vi "Begin.vi"(8 "error in":errorcluster) -> (0 "error out":errorcluster)   [LabVIEW 2015]
doc: "Called before other user functions, this VI is expected to open initial I/O refnums, load in file data, and do all program initialization. Notice that the <B>error out</B> terminal is simply used for data flow. Wiring it to other structures or subVIs ensures that this VI runs first."
uses:
  <vilib>/Rock Robotics/SystemInterfaces/DIO/FPGA_DIOPWMChannel.ctl
  <vilib>/Rock Robotics/WPI/DriverStation/WPI_DriverStationRobotMode2.ctl
  <vilib>/Rock Robotics/WPI/Joystick/WPI_JoystickDeviceEnum.ctl
  <vilib>/Rock Robotics/WPI/Solenoid/WPI_SolenoidChannel.ctl
  <vilib>/Rock Robotics/SystemInterfaces/spilib/spi_bus.ctl
  <vilib>/Rock Robotics/SystemInterfaces/DIO/FPGA_DIOChannel.ctl
  <vilib>/Rock Robotics/WPI/SafetyOutput/WPI_SafetyOutputConfigMenu.ctl
  <vilib>/Rock Robotics/WPI/RobotDrive/WPI_RobotDriveOpen2MotorWithVictor.vi
  Robot Global Data.vi
  <vilib>/Rock Robotics/Network Tables/NT Write String Array.vi
  <vilib>/Rock Robotics/WPI/MotorControl/WPI_MotorControlOpen Talon.vi
  <vilib>/Rock Robotics/WPI/Solenoid/WPI_SolenoidOpenDouble.vi
  <vilib>/Rock Robotics/WPI/Gyro/WPI_GyroXRS450_SPI_Open.vi
  <vilib>/Rock Robotics/WPI/MotorControl/WPI_MotorControlOpen Victor.vi
  <vilib>/Rock Robotics/WPI/Accelerometer/InternalAccelerometer/WPI_AccelerometerInternalOpen.vi
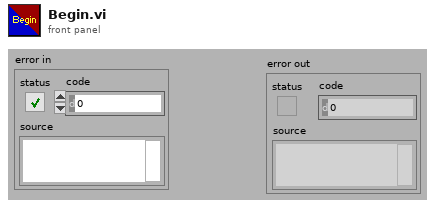
[diagram p1: front panel]
types:
  T1 = typedef "WPI_SafetyOutputConfigMenu.ctl" = enum16{"Enable", "Disable"}
  T2 = typedef "WPI_JoystickDeviceEnum.ctl" = enum16{"USB 0", "USB 1", "USB 2", "USB 3", "USB 4", "USB 5"}
  T3 = typedef "FPGA_DIOChannel.ctl" = enum8{"DIO 0", "DIO 1", "DIO 2", "DIO 3", "DIO 4", "DIO 5", "DIO 6", "DIO 7", "DIO 8", "DIO 9", "DIO MXP 0", "DIO MXP 1", "DIO MXP 2", "DIO MXP 3", "DIO MXP 4", "DIO MXP 5", "DIO MXP 6", "DIO MXP 7", "DIO MXP 8", "DIO MXP 9", "DIO MXP 10", "DIO MXP 11", "DIO MXP 12", "DIO MXP 13", "DIO MXP 14", "DIO MXP 15", "Invalid"}
  T4 = typedef "FPGA_DIOPWMChannel.ctl" = enum8{"PWM 0", "PWM 1", "PWM 2", "PWM 3", "PWM 4", "PWM 5", "PWM 6", "PWM 7", "PWM 8", "PWM 9", "PWM MXP 0", "PWM MXP 1", "PWM MXP 2", "PWM MXP 3", "PWM MXP 4", "PWM MXP 5", "PWM MXP 6", "PWM MXP 7", "PWM MXP 8", "PWM MXP 9", "Invalid"}
  T5 = typedef "WPI_SolenoidChannel.ctl" = enum8{"Solenoid 0", "Solenoid 1", "Solenoid 2", "Solenoid 3", "Solenoid 4", "Solenoid 5", "Solenoid 6", "Solenoid 7", "Invalid"}
  T6 = typedef "spi_bus.ctl" = enum16{"SPI On-Board, CS0", "SPI On-Board, CS1", "SPI On-Board, CS2", "SPI On-Board, CS3", "SPI MXP", "Invalid"}
  T7 = typedef "WPI_DriverStationRobotMode2.ctl" = enum16{"Autonomous Disabled", "Autonomous Enabled", "Teleop Disabled", "Teleop Enabled", "Disconnected", "Finish", "Test Disabled", "Test Enabled", "Emergency Stopped"}
  T8 = typedef "WPI_AccelerometerDevRef.ctl" = cluster{"DevStatus":errorcluster, "Scaling":T9, "Analog Channels":T10, "I2C Bus":T12, "SPI Bus":T6, "Accel Range":T13, "ADXL Axes":T14, "Handle":i32, "Device Address":u8, "Accel Type":enum16{"Analog", "ADXL345 I2C", "ADXL345 SPI", "Internal", "ADXL362 SPI"}}
  T9 = typedef "WPI_AccelerometerScaling.ctl" = cluster{"Gain (VoltsPerG)":dbl, "Center Voltage":dbl}
  T10 = typedef "WPI_AccelerometerAnalogChannels.ctl" = cluster{"X-Axis":T11, "Y-Axis":T11, "Z-Axis":T11}
  T11 = typedef "FPGA_AIChannel.ctl" = enum8{"AI 0", "AI 1", "AI 2", "AI 3", "AI MXP 0", "AI MXP 1", "AI MXP 2", "AI MXP 3", "Invalid"}
  T12 = typedef "i2c_bus.ctl" = enum16{"I2C On-Board", "I2C MXP", "Invalid"}
  T13 = typedef "ADXL345 Range.ctl" = u8
  T14 = typedef "WPI_AccelerometerADXL345 Axes.ctl" = cluster{"X-Axis":bool, "Y-Axis":bool, "Z-Axis":bool}
  T15 = typedef "WPI_DigitalInputDevRef.ctl" = cluster{"DevStatus":errorcluster, "DIO Channel":T3}
  T16 = typedef "WPI_MotorControlDeviceRef.ctl" = cluster{"DeviceStatus":errorcluster, "Type":T17, "PWM":cluster{"PWM Channel":T4, "DeadBand":T18}, "CAN":cluster{"Device Number":u8, "Control Mode":T19, "Semaphore":T20, "Max Vout":dbl, "TalonSRX Control Mode":T21}, "Invert":bool}
  T17 = typedef "WPI_MotorControlType.ctl" = enum16{"PWM", "CAN", "CANTalonSRX"}
  T18 = typedef "WPI_PWMDeadband.ctl" = cluster{"Name":string, "maxPositivePwm":i32, "minPositivePwm":i32, "centerPwm":i32, "maxNegativePwm":i32, "minNegativePwm":i32, "angularRange":u16}
  T19 = typedef "WPI_CANJaguar_ControlMode.ctl" = enum8{"Percent VBus", "Current", "Speed", "Position", "Voltage"}
  T20 = typedef "Semaphore RefNum" = refnum<k1>
  T21 = typedef "WPI_CANTalonSRX_APIControlMode.ctl" = enum8{"Percent VBus", "Speed", "Position", "Slave", "Unchanged / Invalid", "Voltage Compensation", "Current", "Motion Profile"}
  T22 = typedef "WPI_JoystickDevRef.ctl" = cluster{"Device":T2}
  T23 = typedef "WPI_SolenoidDevRef.ctl" = cluster{"DevStatus":errorcluster, "Pneumatics Control Module":u8, "Forward Solenoid Channel":T5, "Reverse Solenoid Channel":T5}
  T24 = typedef "WPI_RobotDriveDevRef.ctl" = cluster{"DevStatus":errorcluster, "Motors[]":T16[], "Square Inputs":bool, "Max Output":dbl}
  T25 = typedef "WPI_GyroDevRef.ctl" = cluster{"DevStatus":errorcluster, "Analog Channel":T11, "Offset":dbl, "Gain (VoltsPerDegree/Second)":dbl, "Gyro Type":enum16{"Analog", "XRS450"}, "Handle":i32, "SPI Bus":T6, "Device Found":bool, "Sample Rate":dbl, "Calibrate On Open":bool}
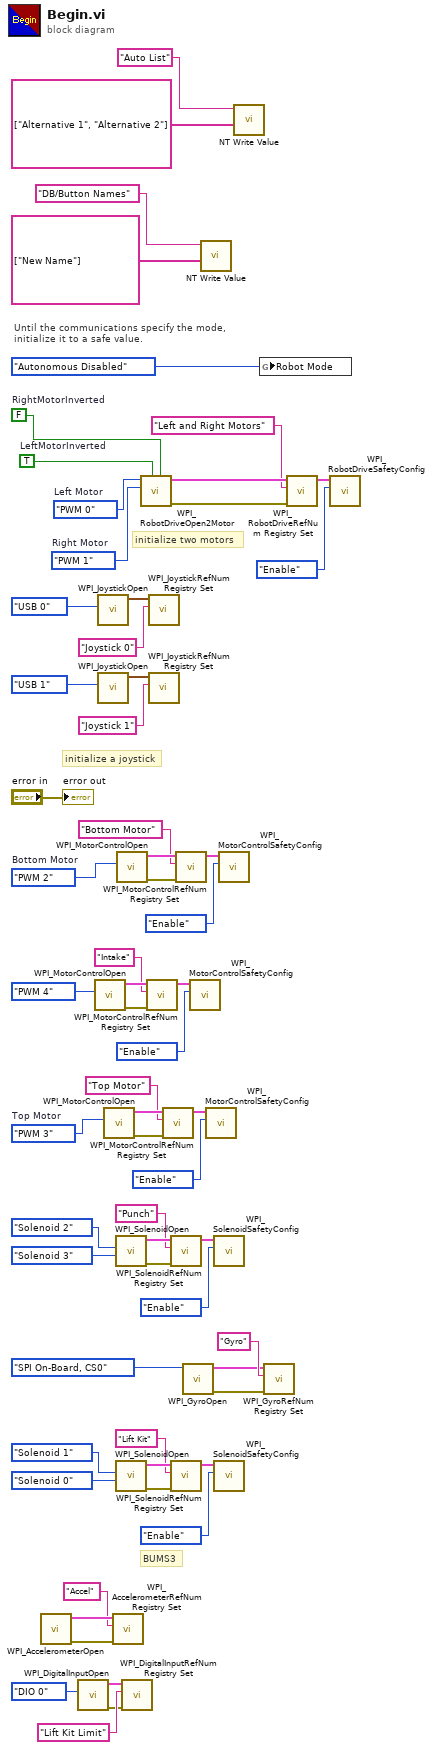
[diagram p0: block diagram]
diagram:
  w45 = FPGA_DIOPWMChannel."PWM 3"  # Top Motor
  w46 = FPGA_DIOPWMChannel."PWM 2"  # Bottom Motor
  w58 = FPGA_DIOPWMChannel."PWM 1"  # Right Motor
  w59 = FPGA_DIOPWMChannel."PWM 0"  # Left Motor
  w63 = TRUE  # LeftMotorInverted
  w64 = FALSE  # RightMotorInverted
  # "BUMS3"
  # "initialize a joystick"
  # "Until the communications specify the mode,\ninitialize it to a safe value."
  # "initialize two motors"
  n1 = call-poly <vilib>:"WPI_AccelerometerOpen.vi"() -> ("error out"=w27:errorcluster, "AccelerometerDevRef"=w30:T8)  [unwired: 10 in]
  n2 = call <vilib>:"WPI_DigitalInputOpen.vi"("DIO Channel"=FPGA_DIOChannel."DIO 0") -> ("error out"=w1:errorcluster, "DigitalInputDevRef"=w17:T15)  [unwired: 9 in]
  n3 = call-poly <vilib>:"WPI_MotorControlOpen.vi"("PWM Channel"=FPGA_DIOPWMChannel."PWM 4") -> ("error out"=w19:errorcluster, "MotorControlDeviceRef"=w22:T16)  [unwired: 9 in]
  n4 = call <vilib>:"WPI_JoystickOpen.vi"("JoystickDevice"=WPI_JoystickDeviceEnum."USB 0") -> ("JoystickDevRef"=w53:T22)  [unwired: 10 in]
  n5 = call <vilib>:"WPI_JoystickOpen.vi"("JoystickDevice"=WPI_JoystickDeviceEnum."USB 1") -> ("JoystickDevRef"=w13:T22)  [unwired: 10 in]
  n6 = call-poly <vilib>:"WPI_MotorControlOpen.vi"("PWM Channel"=w45) -> ("error out"=w39:errorcluster, "MotorControlDeviceRef"=w44:T16)  [unwired: 9 in]
  n7 = call <vilib>:"WPI_AccelerometerRefNum Registry Set.vi"("error in (no error)"=w27, "refnum name"="Accel", "AccelerometerDevRef"=w30) -> ()  [unwired: 7 in, 2 out]
  n8 = call-poly <vilib>:"WPI_SolenoidOpen.vi"("Reverse Solenoid Channel"=WPI_SolenoidChannel."Solenoid 3", "Forward Solenoid Channel"=WPI_SolenoidChannel."Solenoid 2" ("Solenoid Channel")) -> ("error out"=w18:errorcluster, "SolenoidDevRef"=w25:T23)  [unwired: 8 in]
  n9 = call-poly <vilib>:"WPI_SolenoidOpen.vi"("Reverse Solenoid Channel"=WPI_SolenoidChannel."Solenoid 0", "Forward Solenoid Channel"=WPI_SolenoidChannel."Solenoid 1" ("Solenoid Channel")) -> ("error out"=w35:errorcluster, "SolenoidDevRef"=w38:T23)  [unwired: 8 in]
  n10 = call-poly <vilib>:"WPI_MotorControlOpen.vi"("PWM Channel"=w46) -> ("error out"=w40:errorcluster, "MotorControlDeviceRef"=w43:T16)  [unwired: 9 in]
  n11 = call <vilib>:"WPI_DigitalInputRefNum Registry Set.vi"("error in (no error)"=w1, "refnum name"="Lift Kit Limit", "DigitalInputDevRef"=w17) -> ()  [unwired: 7 in, 2 out]
  n12 = call-poly <vilib>:"WPI_RobotDriveOpen2Motor.vi"("Right Motor Inverted"=w64, "Left Motor Inverted"=w63, "Right Motor"=w58, "Left Motor"=w59) -> ("error out"=w60:errorcluster, "RobotDriveDevRef"=w62:T24)  [unwired: 1 in, 5 out]
  n13 = call <vilib>:"WPI_MotorControlRefNum Registry Set.vi"("error in (no error)"=w19, "refnum name"="Intake", "MotorControlDevRef"=w22) -> ("MotorControlDevRef"=w3:T16)  [unwired: 7 in, 1 out]
  n14 = call <vilib>:"WPI_JoystickRefNum Registry Set.vi"("refnum name"="Joystick 0", "JoystickDevRef"=w53) -> ()  [unwired: 8 in, 2 out]
  n15 = call <vilib>:"WPI_JoystickRefNum Registry Set.vi"("refnum name"="Joystick 1", "JoystickDevRef"=w13) -> ()  [unwired: 8 in, 2 out]
  n16 = call <vilib>:"WPI_MotorControlRefNum Registry Set.vi"("error in (no error)"=w39, "refnum name"="Top Motor", "MotorControlDevRef"=w44) -> ("MotorControlDevRef"=w11:T16)  [unwired: 7 in, 1 out]
  n17 = call <vilib>:"WPI_SolenoidRefNum Registry Set.vi"("error in (no error)"=w18, "refnum name"="Punch", "SolenoidDevRef"=w25) -> ("SolenoidDevRef"=w7:T23)  [unwired: 7 in, 1 out]
  n18 = call <vilib>:"WPI_SolenoidRefNum Registry Set.vi"("error in (no error)"=w35, "refnum name"="Lift Kit", "SolenoidDevRef"=w38) -> ("SolenoidDevRef"=w6:T23)  [unwired: 7 in, 1 out]
  n19 = call <vilib>:"WPI_MotorControlRefNum Registry Set.vi"("error in (no error)"=w40, "refnum name"="Bottom Motor", "MotorControlDevRef"=w43) -> ("MotorControlDevRef"=w10:T16)  [unwired: 7 in, 1 out]
  n20 = call-poly <vilib>:"WPI_GyroOpen.vi"("SPI Bus"=spi_bus."SPI On-Board, CS0") -> ("error out"=w29:errorcluster, "GyroDevRef"=w32:T25)  [unwired: 9 in]
  n21 = call <vilib>:"WPI_MotorControlSafetyConfig.vi"("mode"=WPI_SafetyOutputConfigMenu."Enable", "MotorControlDevRef"=w3) -> ()  [unwired: 8 in, 2 out]
  n22 = call-poly <vilib>:"NT Write Value.vi"("String Array"=string[] ["New Name"], "Name"="DB/Button Names") -> ()  [unwired: 9 in, 1 out]
  n23 = call <vilib>:"WPI_MotorControlSafetyConfig.vi"("mode"=WPI_SafetyOutputConfigMenu."Enable", "MotorControlDevRef"=w11) -> ()  [unwired: 8 in, 2 out]
  n24 = call <vilib>:"WPI_SolenoidSafetyConfig.vi"("mode"=WPI_SafetyOutputConfigMenu."Enable", "SolenoidDevRef"=w7) -> ()  [unwired: 8 in, 2 out]
  n25 = call <vilib>:"WPI_SolenoidSafetyConfig.vi"("mode"=WPI_SafetyOutputConfigMenu."Enable", "SolenoidDevRef"=w6) -> ()  [unwired: 8 in, 2 out]
  n26 = call <vilib>:"WPI_MotorControlSafetyConfig.vi"("mode"=WPI_SafetyOutputConfigMenu."Enable", "MotorControlDevRef"=w10) -> ()  [unwired: 8 in, 2 out]
  n27 = call-poly <vilib>:"NT Write Value.vi"("String Array"=string[] ["Alternative 1", "Alternative 2"], "Name"="Auto List") -> ()  [unwired: 9 in, 1 out]
  n28 = global write "Robot Global Data.vi" "Robot Mode"(WPI_DriverStationRobotMode2."Autonomous Disabled" ("Robot Mode")) -> ()
  n29 = call <vilib>:"WPI_GyroRefNum Registry Set.vi"("error in (no error)"=w29, "refnum name"="Gyro", "GyroDevRef"=w32) -> ()  [unwired: 7 in, 2 out]
  n30 = call <vilib>:"WPI_RobotDriveRefNum Registry Set.vi"("error in (no error)"=w60, "refnum name"="Left and Right Motors", "RobotDriveDevRef"=w62) -> ("RobotDriveDevRef"=w57:T24)  [unwired: 1 in, 7 out]
  n31 = call <vilib>:"WPI_RobotDriveSafetyConfig.vi"("mode"=WPI_SafetyOutputConfigMenu."Enable", "RobotDriveDevRef"=w57) -> ()  [unwired: 8 in, 2 out]
  "error out" <- "error in"
